vi "Ball ROI (SubVI).vi"(5 "ROI Descriptor COLOR Mask":T1={"Global Rectangle"=[109, 72, 345, 284], "Contours"=[{"ID"=enum."External", "Type"=3, "Coordinates"=[109, 72, 345, 284]}]} {"Contours"."Type" items=["No Selection", "Point", "Line", "Rectangle", "Oval", "Polygon", "Freehand Region", "Annulus", "Unused2", "Unused3", "Broken Line", "Freehand Line", "Rotated Rectangle"]}, 6 "divider (circle)":dbl=1.0, 8 "curY":dbl, 9 "curX":dbl, 10 "Boolean":bool, 11 "Radius":dbl) -> (0 "x1":i32, 1 "y0":i32, 2 "x0":i32, 3 "ROI Descriptor COLOR Mask out":T1={"Global Rectangle"=[109, 72, 345, 284], "Contours"=[{"ID"=enum."External", "Type"=3, "Coordinates"=[109, 72, 345, 284]}]} {"Contours"."Type" items=["No Selection", "Point", "Line", "Rectangle", "Oval", "Polygon", "Freehand Region", "Annulus", "Unused2", "Unused3", "Broken Line", "Freehand Line", "Rotated Rectangle"]}, 4 "y1":i32)   [LabVIEW 2017]
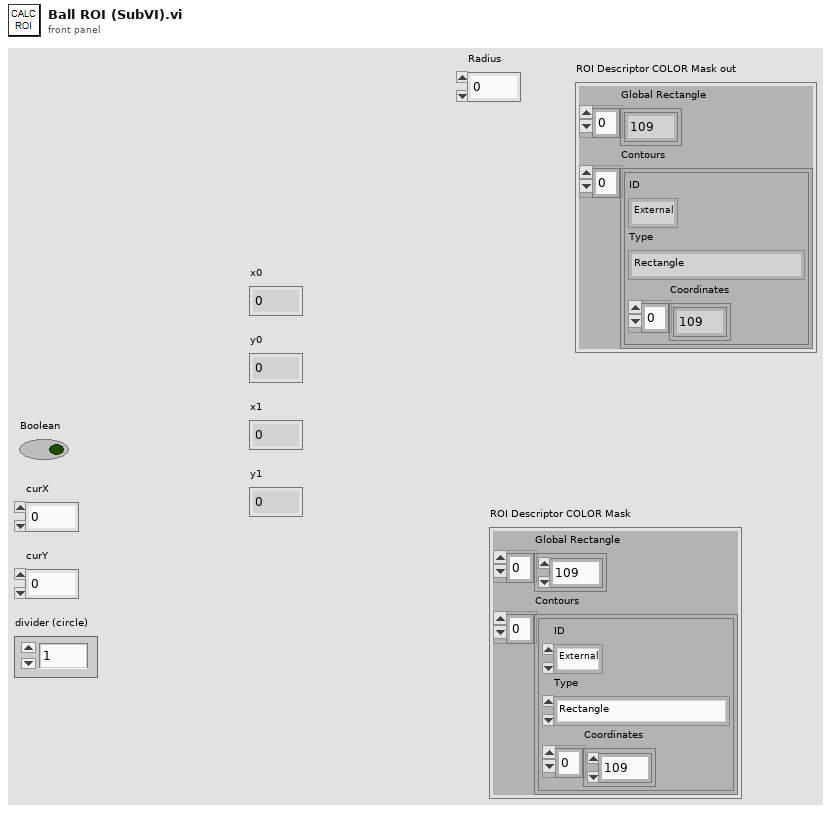
[diagram p1: front panel]
types:
  T1 = cluster{"Global Rectangle":i32[], "Contours":cluster{"ID":enum32{"External", "Internal"}, "Type":u32, "Coordinates":i32[]}[]}
  T2 = cluster{"ID":enum32{"External", "Internal"}, "Type":u32, "Coordinates":i32[]}[]
  T3 = cluster{"ID":enum32{"External", "Internal"}, "Type":u32, "Coordinates":i32[]}
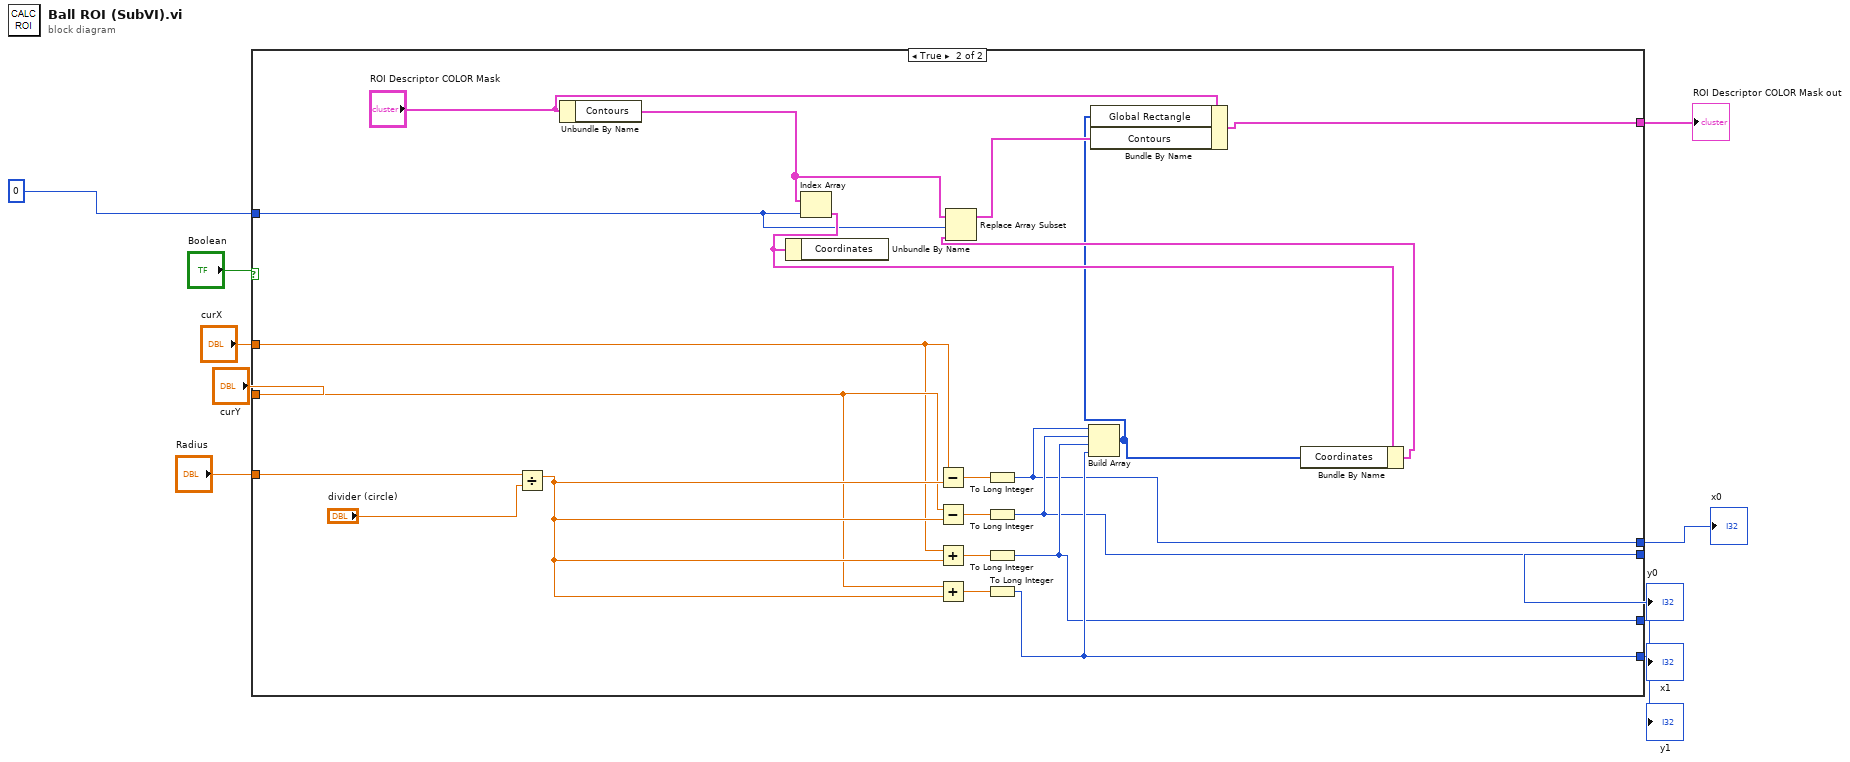
[diagram p0: block diagram]
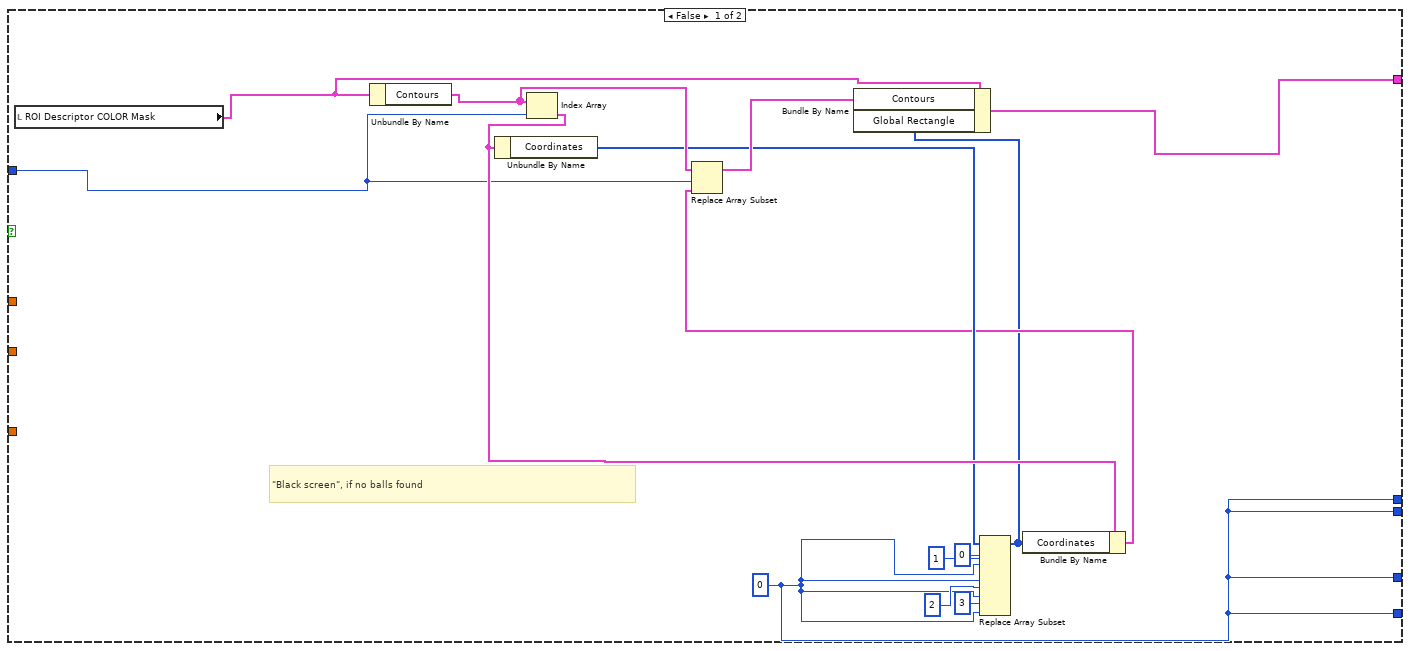
[diagram p2: hidden frame]
diagram:
  n1 = case shown="True" "Boolean" {
    tunnel: 0 ("Ball index") -> [w14 w34]
    tunnel: [w19 w31] -> w5
    tunnel: [w19 w30] -> w6
    tunnel: [w19 w28] -> w7
    tunnel: [w19 w29] -> w8
    tunnel: "curY" -> [_ w38]
    tunnel: "curX" -> [_ w37]
    tunnel: "Radius" -> [_ w26]
    tunnel: [w11 w25] -> w1
    frame False {
      w19 = 0 ("index")
      # "\"Black screen\", if no balls found"
      n2 = local read "ROI Descriptor COLOR Mask"() -> (w15:T1)
      n3 = Unbundle By Name(w15) -> ("Contours"=w18:T2)
      n4 = Index Array(array=w18, index=w14) -> (element=w17:T3)
      n5 = Unbundle By Name(w17) -> ("Coordinates"=w16:i32[])
      n6 = Replace Array Subset(array=w16, new element #1=w19, index #1=0 ("index"), new element #2=w19, index #2=1 ("index"), new element #3=w19, index #3=2 ("index"), new element #4=w19, index #4=3 ("index")) -> (w12:i32[])
      n7 = Bundle By Name(cluster=w17, "Coordinates"=w12) -> (w13:T3)
      n8 = Replace Array Subset(array=w18, new element=w13, index=w14) -> (w20:T2)
      n9 = Bundle By Name(cluster=w15, "Contours"=w20, "Global Rectangle"=w12) -> (w11:T1)
    }
    frame True {
      n10 = Divide(x=w26, y="divider (circle)") -> (x/y=w41:dbl)
      n11 = Unbundle By Name("ROI Descriptor COLOR Mask") -> ("Contours"=w39:T2)
      n12 = Index Array(array=w39, index=w34) -> (element=w40:T3)
      n13 = Unbundle By Name(w40) -> ()  [unwired: 1 out]
      n14 = Subtract(x=w37, y=w41) -> (x-y=w45:dbl)
      n15 = Subtract(x=w38, y=w41) -> (x-y=w44:dbl)
      n16 = Add(x=w37, y=w41) -> (x+y=w42:dbl)
      n17 = Add(x=w38, y=w41) -> (x+y=w43:dbl)
      n18 = To Long Integer(number=w45) -> (32bit integer=w28:i32)
      n19 = To Long Integer(number=w44) -> (32bit integer=w29:i32)
      n20 = To Long Integer(number=w42) -> (32bit integer=w30:i32)
      n21 = To Long Integer(number=w43) -> (32bit integer=w31:i32)
      n22 = Build Array(w28, w29, w30, w31) -> (w27:i32[])
      n23 = Bundle By Name(cluster=w40, "Coordinates"=w27) -> (w33:T3)
      n24 = Replace Array Subset(array=w39, new element=w33, index=w34) -> (w35:T2)
      n25 = Bundle By Name(cluster="ROI Descriptor COLOR Mask", "Global Rectangle"=w27, "Contours"=w35) -> (w25:T1)
    }
  }
  "y0" <- w8
  "x0" <- w7
  "x1" <- w6
  "y1" <- w5
  "ROI Descriptor COLOR Mask out" <- w1
